vi "FindControlByName.vi"(3 "error in (no error)":errorcluster, 4 "control name":string, 5 "vi refnum":refnum<vi>) -> (0 "error out":errorcluster, 2 "control refnum":refnum<vi>)   [LabVIEW 2015]
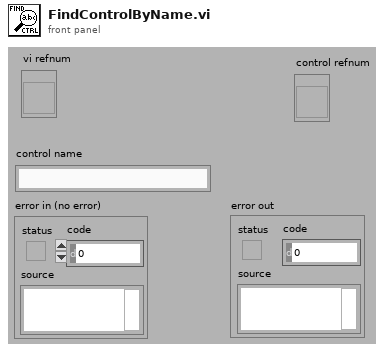
[diagram p1: front panel]
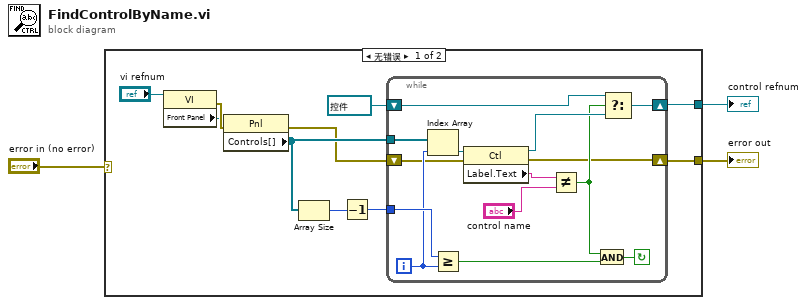
[diagram p0: block diagram]
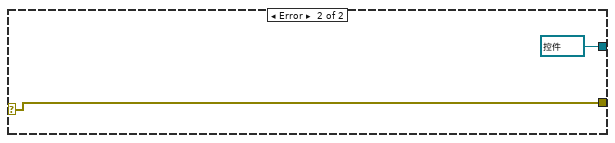
[diagram p2: hidden frame]
diagram:
  n1 = case shown="无错误" "error in (no error)" {
    selector: "error in (no error)" -> [_ w29]
    tunnel: [w7 refnum<vi> refnum ("dup reference")] -> w3
    tunnel: [w4 w29] -> w2
    frame No Error {
      n2 = property class="VI"(reference="vi refnum") -> (error out=w12:errorcluster, "Front Panel"=w11:refnum<vi>)  [unwired: 1 in, 1 out]
      n3 = property class="Pnl"(reference=w11, error in=w12) -> (error out=w5:errorcluster, "Controls[]"=w9:refnum<vi>[])  [unwired: 1 out]
      n4 = Array Size(array=w9) -> (size(s)=w10:i32)
      n5 = Decrement(x=w10) -> (x-1=w6:i32)
      n6 = while {
        tunnel: w6 -> [w27]
        tunnel: w9 -> [w26]
        shift-right: [w21] -> w7
        shift-left: refnum<vi> refnum ("dup reference") -> [w20]
        shift-right: [w14] -> w4
        shift-left: w5 -> [w15]
        i -> [w25]
        stop <- w18 continue-if-true
        n7 = Index Array(array=w26, index=w25) -> (element=w24:refnum<vi>)
        n8 = Greater Or Equal?(x=w27, y=w25) -> (x >= y?=w16:bool)
        n9 = property class="Ctl"(reference=w24, error in=w15) -> (reference out=w19:refnum<vi>, error out=w14:errorcluster, "Label.Text"=w23:string)
        n10 = Not Equal?(x=w23, y="control name") -> (x != y?=w17:bool)
        n11 = And(x=w17, y=w16) -> (x .and. y?=w18:bool)
        n12 = Select(t=w20, s=w17, f=w19) -> (s? t:f=w21:refnum<vi>)
      }
    }
    frame Error {
    }
  }
  "control refnum" <- w3
  "error out" <- w2
